vi "ReadFromDAQ_Wfm.vi"() -> ()   [LabVIEW 2025]
uses:
  <vilib>/DAQmx/read.llb/DAQmx Read (Analog 1D Wfm NChan NSamp).vi
  <vilib>/DAQmx/create/channels.llb/DAQmx Create Channel (AI-Voltage-Basic).vi
  <vilib>/DAQmx/configure/timing.llb/DAQmx Timing (Sample Clock).vi
  <vilib>/DAQmx/miscellaneous.llb/DAQmx Fill In Error Info.vi
panel:
  out "History Data 2":waveform(dbl)[][](array[waveform])
  out "Waveform Graph":waveform(dbl)[](graph)
  in  "error in":errorcluster
  in  "clear chart":bool
  in  "clock settings":T1={"sample mode"=10178, "samples per channel"=1000, "rate"=1000.0} {"sample mode" items=["Finite Samples"=10178, "Continuous Samples"=10123, "Hardware Timed Single Point"=12522]}
  in  "channel settings":T2={"max value"=5.0, "min value"=-5.0, "physical channels"="Dev1/ai2", "input terminal configuration"=-1, "units"=10348} {"input terminal configuration" items=["Default"=-1, "RSE"=10083, "NRSE"=10078, "Differential"=10106, "Pseudodifferential"=12529]; "units" items=["Volts"=10348, "From Custom Scale"=10065]}
  out "data":waveform(dbl)[](graph) caption="Waveform Chart"
  out "error out":errorcluster
  in  "stop":bool
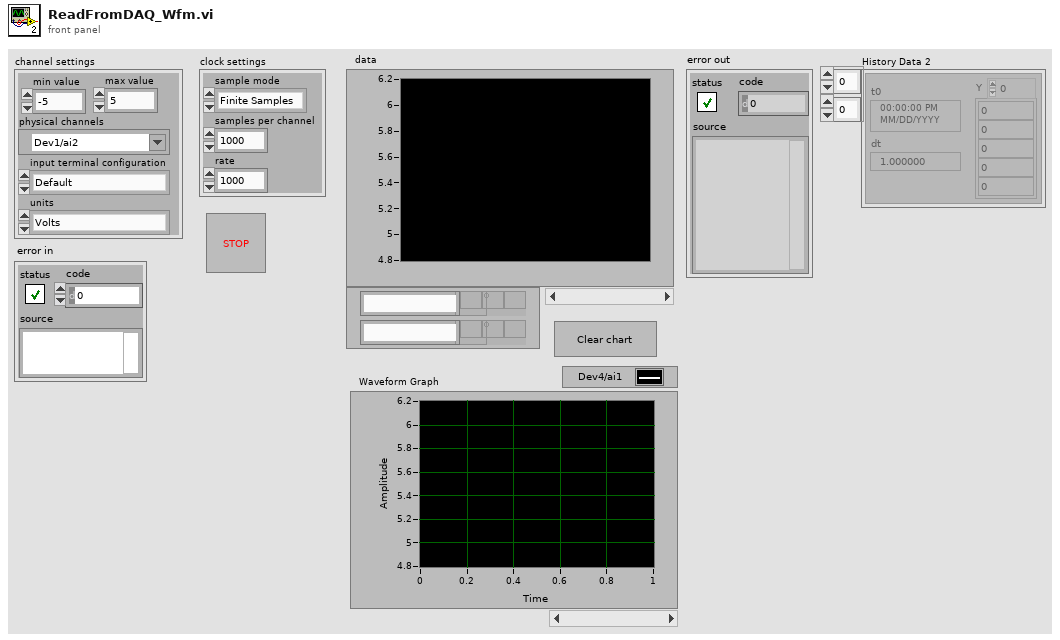
[diagram p1: front panel]
types:
  T1 = cluster{"sample mode":i32, "samples per channel":i32, "rate":dbl}
  T2 = cluster{"max value":dbl, "min value":dbl, "physical channels":tag, "input terminal configuration":i32, "units":i32}
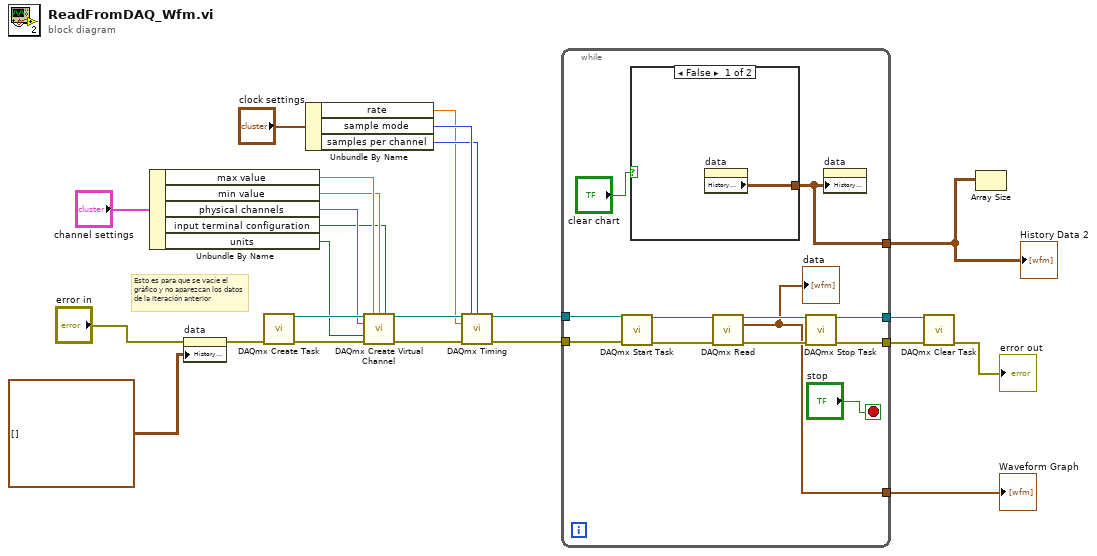
[diagram p0: block diagram]
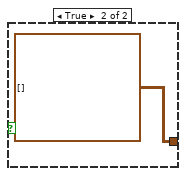
[diagram p2: hidden frame]
diagram:
  # "Esto es para que se vacíe el gráfico y no aparezcan los datos de la iteración anterior"
  n1 = Unbundle By Name("channel settings") -> ("max value"=w10:dbl, "min value"=w9:dbl, "physical channels"=w11:tag, "input terminal configuration"=w8:i32, "units"=w7:i32)
  n2 = property on="data" class="WFChart (strict)"(error in="error in", "History Data"=waveform(dbl)[][] [] ("History Data 2")) -> (error out=w4:errorcluster)  [unwired: 1 in, 1 out]
  n3 = call <vilib>:"DAQmx Create Task.vi"("error in"=w4) -> ("task out"=w23:refnum<k21>, "error out"=w22:errorcluster)  [unwired: 13 in]
  n4 = Unbundle By Name("clock settings") -> ("rate"=w6:dbl, "sample mode"=w14:i32, "samples per channel"=w13:i32)
  n5 = call-poly <vilib>:"DAQmx Create Virtual Channel.vi"("task in"=w23, "maximum value"=w10, "minimum value"=w9, "input terminal configuration"=w8, "physical channels"=w11, "units"=w7, "error in"=w22) -> ("task out"=w24:refnum<k21>, "error out"=w21:errorcluster)  [unwired: 7 in]
  n6 = call-poly <vilib>:"DAQmx Timing.vi"("task/channels in"=w24, "sample mode"=w14, "samples per channel"=w13, "rate"=w6, "error in"=w21) -> ("task out"=w20:refnum<k21>, "error out"=w19:errorcluster)  [unwired: 9 in]
  n7 = while {
    tunnel: w20 -> [w31]
    tunnel: w19 -> [w30]
    tunnel: [w29] -> w18
    tunnel: [w28] -> w17
    tunnel: [w26] -> w2
    tunnel: [w25] -> w1
    stop <- "stop" stop-if-true
    n8 = call <vilib>:"DAQmx Start Task.vi"("task/channels in"=w31, "error in"=w30) -> ("task out"=w36:refnum<k21>, "error out"=w34:errorcluster)  [unwired: 12 in]
    n9 = case shown="False" "clear chart" {
      tunnel: [w37 waveform(dbl)[][] [] ("History Data 2")] -> w26
      frame False {
        n10 = property on="data" class="WFChart (strict)"() -> ("History Data"=w37:waveform(dbl)[][])  [unwired: 2 in, 2 out]
      }
      frame True {
      }
    }
    n11 = call-poly <vilib>:"DAQmx Read.vi"("task/channels in"=w36, "error in"=w34) -> ("task out"=w35:refnum<k21>, "data"=w25:waveform(dbl)[], "error out"=w33:errorcluster)  [unwired: 11 in]
    "data" <- w25
    n12 = call <vilib>:"DAQmx Stop Task.vi"("task/channels in"=w35, "error in"=w33) -> ("task out"=w29:refnum<k21>, "error out"=w28:errorcluster)  [unwired: 12 in]
    n13 = property on="data" class="WFChart (strict)"("History Data"=w26) -> ()  [unwired: 2 in, 2 out]
  }
  "History Data 2" <- w2
  "Waveform Graph" <- w1
  n14 = call <vilib>:"DAQmx Clear Task.vi"("task in"=w18, "error in"=w17) -> ("error out"=→"error out":errorcluster)  [unwired: 13 in]
  n15 = Array Size(array=w2) -> ()  [unwired: 1 out]
